vi "Get State.vi"(8 "error in":errorcluster, 9 "timeout (-1)":i32=-1, 11 "Standard Engine Runtime in":refnum<class "Standard Engine Runtime.lvclass">) -> (0 "error out":errorcluster, 2 "Engine State":T1=enum."Closed", 3 "Standard Engine Runtime out":refnum<class "Standard Engine Runtime.lvclass">)   [LabVIEW 2013, in "Standard Engine Runtime.lvclass"]
doc: "Returns the current execution state of the engine."
uses:
  Standard Engine Runtime.lvclass
  <vilib>/NI/Module Execution Interface/Engine Runtime/Execution States.ctl
  Standard Engine Runtime.lvclass/Standard Engine Runtime.ctl
  <vilib>/NI/Module Execution Interface/Engine Runtime/Engine Runtime Interface.lvclass
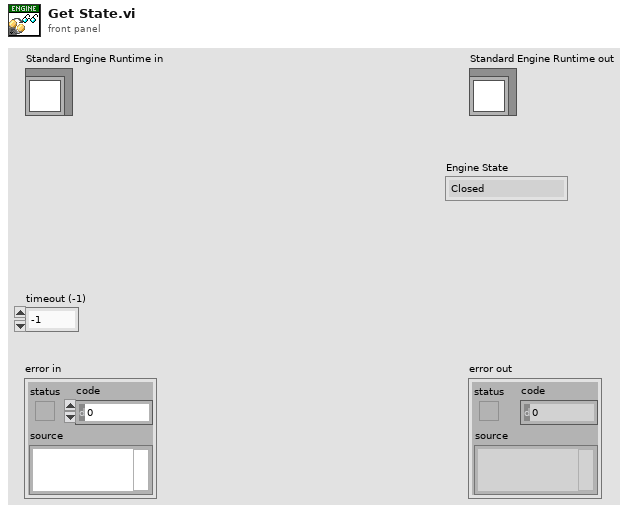
[diagram p1: front panel]
types:
  T1 = typedef "Engine Runtime Interface.lvclass/Execution States.ctl" = enum16{"Initializing", "Paused (Initialized)", "Running", "Set Safe Outputs", "Uninitializing", "Stopped (Uninitialized)", "Error (Uninitialized)", "Safe State (Uninitialized)", "Closed"}
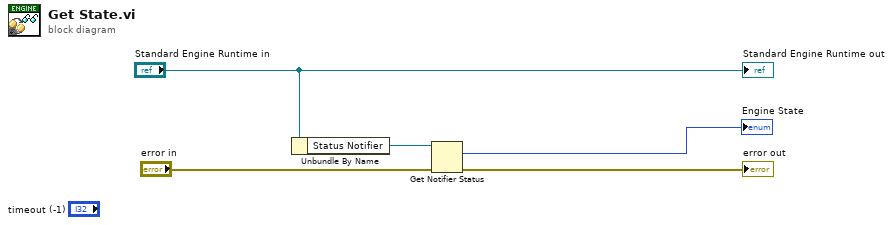
[diagram p0: block diagram]
diagram:
  n1 = Unbundle By Name("Standard Engine Runtime in") -> ("Status Notifier"=w4:refnum<notifier>)
  n2 = Get Notifier Status(notifier=w4, error in (no error)="error in") -> (current notification=→"Engine State":T1, error out=→"error out":errorcluster)  [unwired: 3 out]
  "Standard Engine Runtime out" <- "Standard Engine Runtime in"
